vi "ex4-3.vi"() -> ()   [LabVIEW 2009]
uses:
  <vilib>/NXT/Dual Mode Library/Waits/Wait_Num.vi
  <vilib>/NXT/Dual Mode Library/Motors/MotorOn.vi
panel:
  out "Numeric":dbl
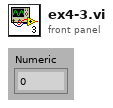
[diagram p1: front panel]
types:
  T1 = typedef "LVHSConnector.ctl" = cluster{"error":errorcluster, "address":string, "NXT #":i32, "Show Error":bool, "Connection":u16}
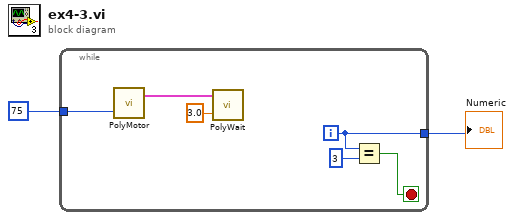
[diagram p0: block diagram]
diagram:
  n1 = while {
    tunnel: i8 75 ("Power (75)") -> [w8]
    tunnel: [w3] -> w1
    i -> [w3]
    stop <- w4 stop-if-true
    n2 = call-poly <vilib>:"PolyMotor.vi"("Power (75)"=w8) -> ("NXT"=w7:T1)  [unwired: 3 in]
    n3 = call-poly <vilib>:"PolyWait.vi"("Time (1 sec)"=sgl 3.0, "NXT"=w7) -> ()  [unwired: 2 in, 1 out]
    n4 = Equal?(x=w3, y=3) -> (x = y?=w4:bool)
  }
  "Numeric" <- w1
